vi "PH_Beckhoff_PPMA-Rods.destructor.vi"(0 "i ref in":refnum<vi>, 5 "error in(no error)":errorcluster) -> (19 "error out":errorcluster)   [LabVIEW 2014, in "PH_Beckhoff_PPMA-Rods.lvlib"]
doc: "This is the destructor of a class.\n\nLicense Agreement for this software:\n\nCopyright (C)\nGesellschaft für Schwerionenforschung, GSI\nPlanckstr. 1\n64291 Darmstadt\nGermany\n\nContact: D.Beck@gsi.de \n\nThis program is free software; you can redistribute it and/or modify it under the terms of the \nGNU General Public License as published by the Free Software Foundation; either version 2 of \nthe license, or (at your option) any later version.\n\nThis program is distributed in the hope that it will be useful, but WITHOUT ANY WARRANTY; \nwithout even the implied warranty of MERCHANTABILITY or FITNESS FOR A PARTICULAR PURPOSE. See the GNU General License for more details (http://www.gnu.org).\n\nGesellschaft für Schwerionenforschung, GSI\nPlanckstr. 1, 64291 Darmstadt, Germany\nFor all questions and ideas contact: M.Richter@gsi.de, H.Brand@gsi.de or D.Beck@gsi.de.\nLast update: 16-JUN-2004"
uses:
  PH_Beckhoff_PPMA-Rods.lvlib
  PH_Beckhoff/PH_Beckhoff.lvlib
  lib.lib/DimLVEvent/LVDimInterface/LVDimInterface.lvlib
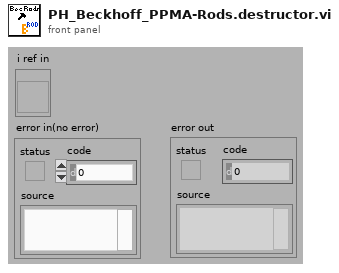
[diagram p1: front panel]
types:
  T1 = typedef "PH_Beckhoff_PPMA-Rods.lvlib/PH_Beckhoff_PPMA-Rods.i attribute.ctl" = cluster{"Input Up GUI Refs":refnum<vi>[], "Output GUI Refs":cluster{"Rod A up":refnum<vi>, "Rod B up":refnum<vi>, "Warnlamp orange":refnum<vi>, "Warnlamp green":refnum<vi>}, "States":cluster{"GUI Ref":refnum<vi>, "Status":T2, "Service ID":i32}[], "Input GUI Refs":cluster{"earth ok":refnum<vi>, "door locked K1":refnum<vi>, "door locked K2":refnum<vi>, "valve closed":refnum<vi>}}
  T2 = typedef "PH_StatusHandler.lvlib/PH_StatusHandler.Status.ctl" = i16
  T3 = enum16{"SetAttribute", "GetAttribute", "CreateAttribute", "DestroyAttribute", "DestroyAllAtributes"}
  T4 = cluster{"GUI Ref":refnum<vi>, "Status":T2, "Service ID":i32}[]
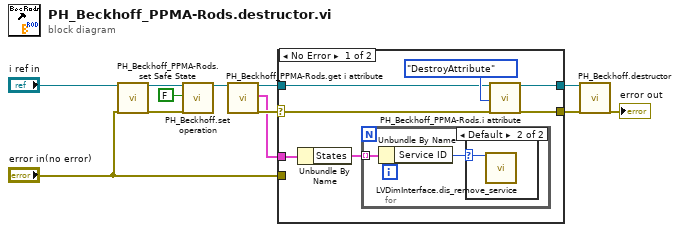
[diagram p0: block diagram]
diagram:
  n1 = call "PH_Beckhoff_PPMA-Rods.set Safe State.vi"("i ref in"="i ref in", "error in"="error in(no error)") -> ("i ref out"=w3:refnum<vi>, "error out"=w4:errorcluster)  [unwired: 16 in]
  n2 = call "PH_Beckhoff.set operation.vi"("VI in"=w3, "operation?"=FALSE, "error in (no error)"=w4) -> ("VI out"=w2:refnum<vi>)  [unwired: 15 in, 1 out]
  n3 = call "PH_Beckhoff_PPMA-Rods.get i attribute.vi"("i ref in"=w2) -> ("i ref out"=w11:refnum<vi>, "i attribute"=w9:T1, "error out"=w10:errorcluster)  [unwired: 16 in]
  n4 = case shown="No Error" w10 {
    selector: w10 -> [w13 _]
    tunnel: [w19 w23] -> w12
    tunnel: w11 -> [w14 w24]
    tunnel: [w18 w24] -> w8
    tunnel: w9 -> [w17 _]
    tunnel: "error in(no error)" -> [_ w23]
    frame No Error {
      n5 = Unbundle By Name(w17) -> ("States"=w16:T4)
      n6 = for {
        tunnel: w16 -> [w21] mode=indexing
        n7 = Unbundle By Name(w21) -> ("Service ID"=w20:i32)
        n8 = case shown="Default" w20 {
          selector: w20 -> [_ w22]
          frame -1 {
          }
          frame Default {
            n9 = call "LVDimInterface.dis_remove_service.vi"("my_serviceID"=w22) -> ()  [unwired: 18 in, 1 out]
          }
        }
      }
      n10 = call "PH_Beckhoff_PPMA-Rods.i attribute.vi"("VI Refnum"=w14, "Action"=T3."DestroyAttribute", "error in (no error)"=w13) -> ("VI Refnum out"=w18:refnum<vi>, "error out"=w19:errorcluster)  [unwired: 14 in, 1 out]
    }
    frame Error {
    }
  }
  n11 = call "PH_Beckhoff.destructor.vi"("i ref in"=w8, "error in(no error)"=w12) -> ("error out"=→"error out":errorcluster)  [unwired: 17 in]
